vi "InstrumentSelectionByName.vi"(8 "error in (no error)":errorcluster, 9 "Verify GPIB address":bool, 11 "Instrument name IN":string) -> (0 "error out":errorcluster, 1 "Instrument name OUT":string, 2 "LCR":refnum<class "LCRControl.lvclass">, 3 "Supply":refnum<class "SupplyControl.lvclass">, 4 "Switching":refnum<class "Switching.lvclass">, 5 "Multimeter":refnum<class "MultimeterControl.lvclass">)   [LabVIEW 2018, in "InstrControl.lvclass"]
uses:
  InstrControl.lvclass
  SupplyControl/SupplyControl.lvclass
  LCRControl/LCRControl.lvclass
  MultimeterControl/MultimeterControl.lvclass
  Switching/Switching.lvclass
  ArduinoControl/ArduinoControl.lvclass
  SupplyControl/Keithley 2657/KE2657A.lvclass
  C:/Users/itk/Documents/itk-strip-sensor-qc/InstrControl/SupplyControl/SupplyControl.lvclass
  C:/Users/itk/Documents/itk-strip-sensor-qc/InstrControl/InstrControl.lvclass
  LCRControl/WK6440B/WK6440B.lvclass
  C:/Users/itk/Documents/itk-strip-sensor-qc/InstrControl/LCRControl/LCRControl.lvclass
  SupplyControl/Keithley 236 & 237/KE236.lvclass
  MultimeterControl/Keithley 2000/KE2000.lvclass
  C:/Users/itk/Documents/itk-strip-sensor-qc/InstrControl/MultimeterControl/MultimeterControl.lvclass
  Switching/Pickering/Pickering.lvclass
  C:/Users/itk/Documents/itk-strip-sensor-qc/InstrControl/Switching/Switching.lvclass
  Switching/PickeringPrague/PickeringPrague.lvclass
  InstrumentSetup.vi
  SupplyControl/Keithley 6517/KE6517.lvclass
  SupplyControl/Keithley 2410/KE2410.lvclass
  SupplyControl/Keithley 487/KE487.lvclass
  LCRControl/WK6425/WK6425.lvclass
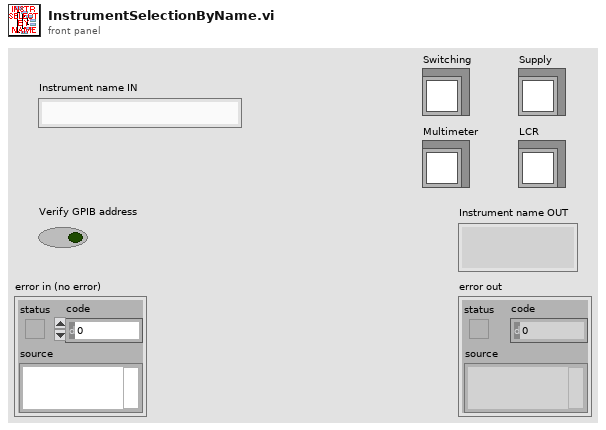
[diagram p1: front panel]
types:
  T1 = cluster{"VISA address":refnum<visa-resource-name>, "T sensor":enum16{"SHT", "DS"}, "Arduino":refnum<class "ArduinoControl.lvclass">}
  T2 = cluster{"KE 2410":cluster{"Instrument name":string, "GPIB address":string, "Instrument type":u16}, "KE 6517":cluster{"Instrument name":string, "GPIB address":string, "Instrument type":u16}, "KE 487":cluster{"Instrument name":string, "GPIB address":string, "Instrument type":u16}, "KE 487_2":cluster{"Instrument name":string, "GPIB address":string, "Instrument type":u16}, "KE 236":cluster{"Instrument name":string, "GPIB address":string, "Instrument type":u16}, "WK 6440B":cluster{"Instrument name":string, "GPIB address":string, "Instrument type":u16}, "WK 6425":cluster{"Instrument name":string, "GPIB address":string, "Instrument type":u16}, "Pickering Matrix":cluster{"Instrument name":string, "GPIB address":string, "Instrument type":u16}, "KE 2000":cluster{"Instrument name":string, "GPIB address":string, "Instrument type":u16}, "KE 2657A":cluster{"Instrument name":string, "GPIB address":string, "Instrument type":u16}, "Prague Pickering Matrix":cluster{"Instrument name":string, "GPIB address":string, "Instrument type":u16}}
  T3 = cluster{"Instrument name":string, "GPIB address":string, "Instrument type":u16}[]
  T4 = cluster{"Current Limit":sgl, "KE2410":refnum<class "KE2410.lvclass">}
  T5 = cluster{"Current Limit":u16, "KE6517":refnum<class "KE6517.lvclass">}
  T6 = cluster{"Compliance":u16, "Range:":u16, "KE487":refnum<class "KE487.lvclass">}
  T7 = cluster{"Current Limit":sgl, "Compliance":u16, "Range:":u16, "KE2657A":refnum<class "KE2657A.lvclass">}
  T8 = cluster{"current \ncompliance level":dbl, "compliance/\nmeasurement range (auto:0)":u16, "KE236":refnum<class "KE236.lvclass">}
  T9 = cluster{"RC Configuration":u16, "AC amplitude [V]":dbl, "AC frequency [Hz]":i32, "WK6440B":refnum<class "WK6440B.lvclass">}
  T10 = cluster{"RC Configuration":u16, "AC amplitude [V]":dbl, "AC frequency [Hz]":i32, "WK6425":refnum<class "WK6425.lvclass">}
  T11 = cluster{"Range":u16, "Range Value":dbl, "Function":u16, "KE2000":refnum<class "KE2000.lvclass">}
  T12 = cluster{"Matrix address":string, "Mux1 address":string, "Mux2 address":string, "Matrix used?":bool, "Pickering":refnum<class "Pickering.lvclass">, "Matrix X Channels":cluster{"Bias Supply / SMU LO":i32, "Bias Supply / SMU HI":i32, "CV Box LO":i32, "CV Box HI":i32, "CV Box LO IN":i32, "CV Box HI IN":i32, "Volt meter LO":i32, "Volt meter HI":i32, "Mux1 C1":i32, "Mux1 C2":i32, "Mux2 C1":i32, "Mux2 C2":i32}}
  T13 = cluster{"Matrix address":string, "Mux1 address":string, "Mux2 address":string, "Matrix used?":bool, "Matrix X Channels":cluster{"LCR LO":i32, "LCR HI":i32, "SMU LO":i32, "SMU HI":i32, "GND":i32}, "Matrix Y Channels":cluster{"Flying Probe":i32, "Needle":i32}, "PickeringPrague.lvclass":refnum<class "PickeringPrague.lvclass">}
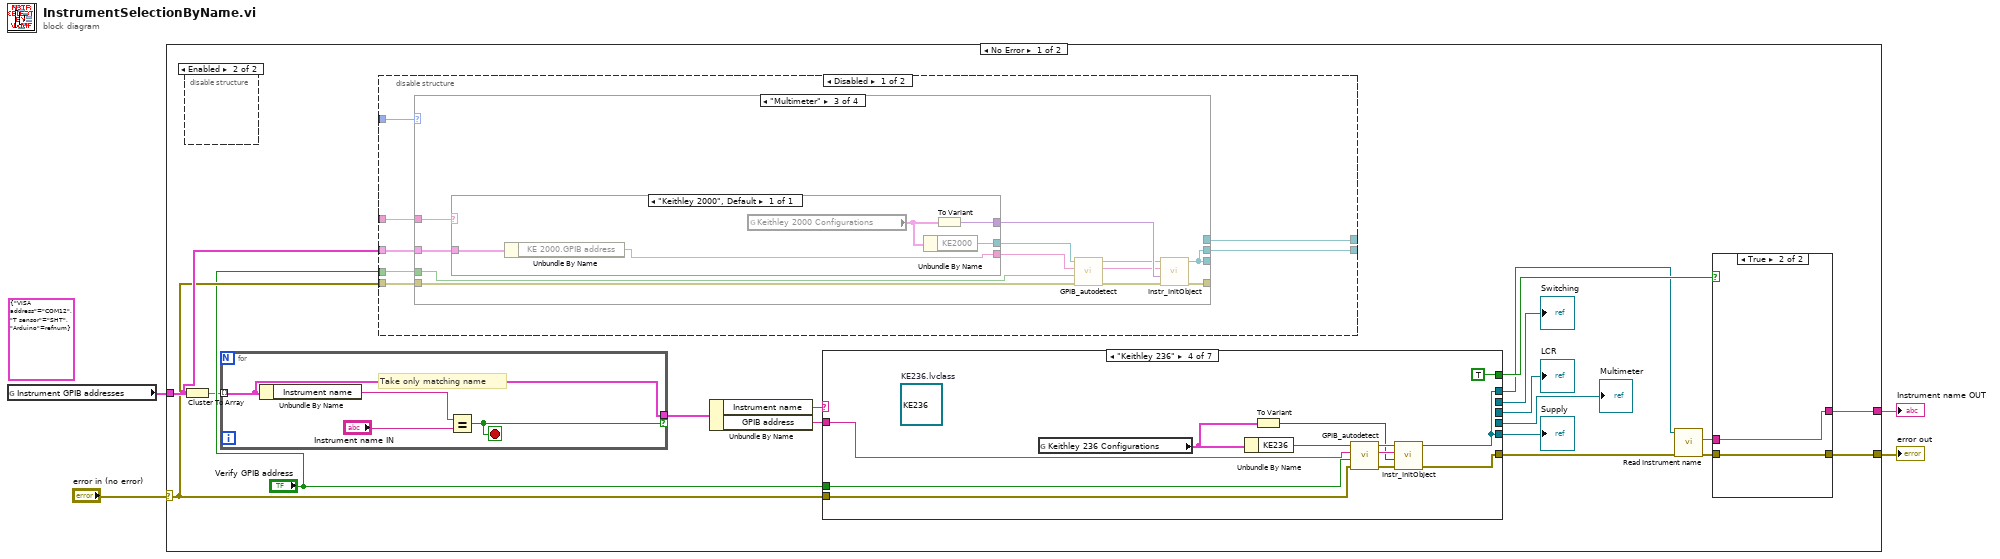
[diagram p0: block diagram]
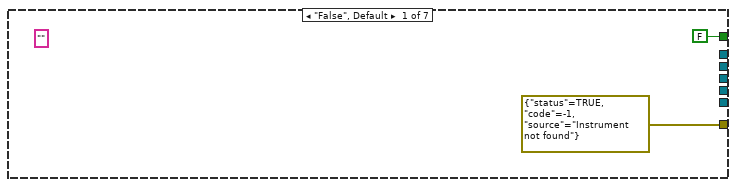
[diagram p2: hidden frame]
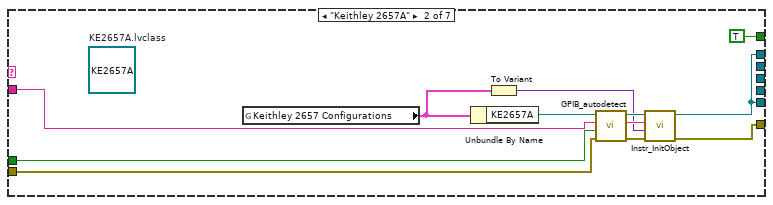
[diagram p3: hidden frame]
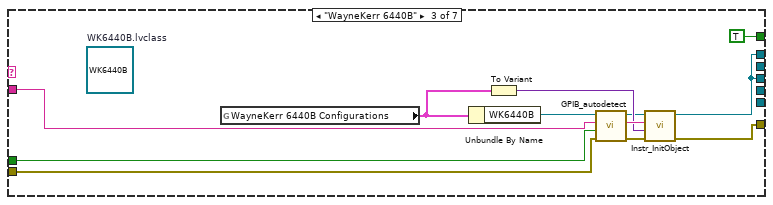
[diagram p4: hidden frame]
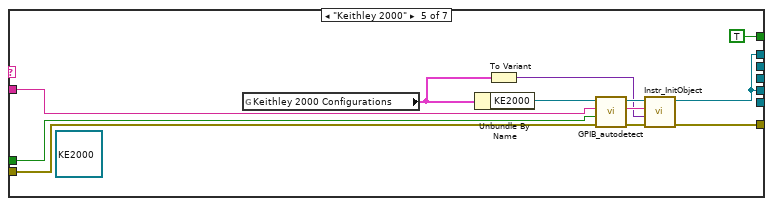
[diagram p5: hidden frame]
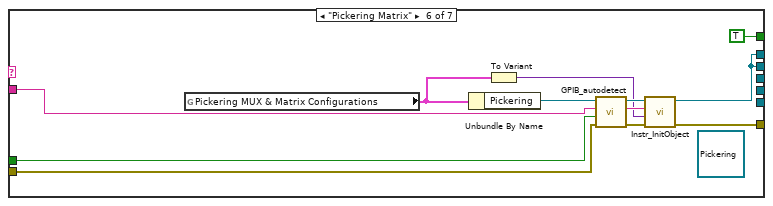
[diagram p6: hidden frame]
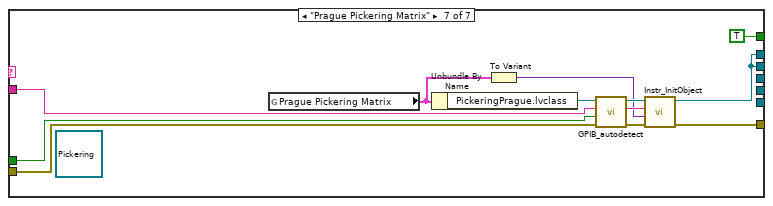
[diagram p7: hidden frame]
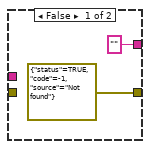
[diagram p8: hidden frame]
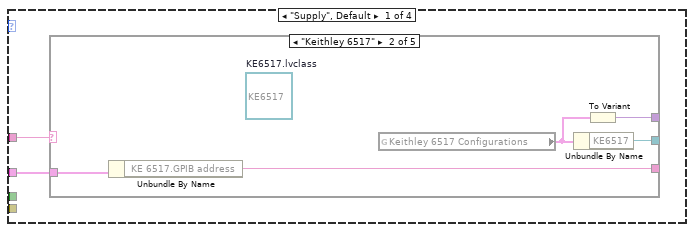
[diagram p9: hidden frame]
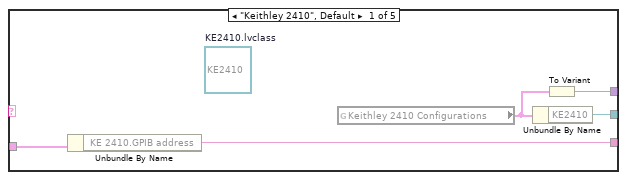
[diagram p10: hidden frame]
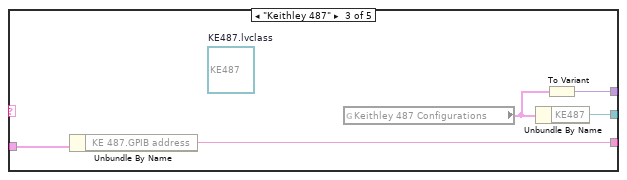
[diagram p11: hidden frame]
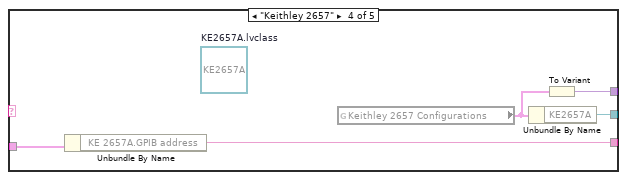
[diagram p12: hidden frame]
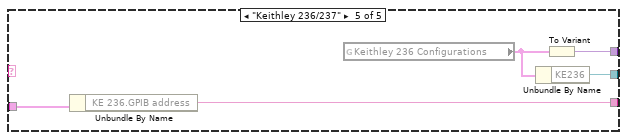
[diagram p13: hidden frame]
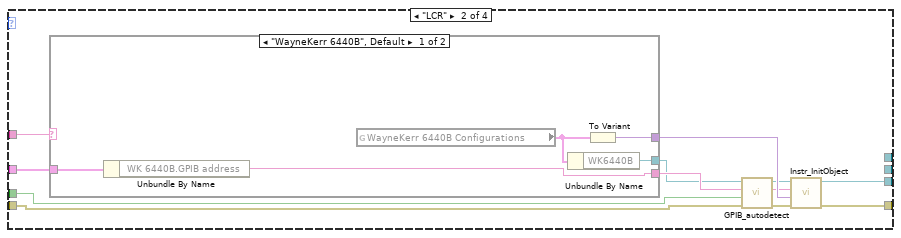
[diagram p14: hidden frame]
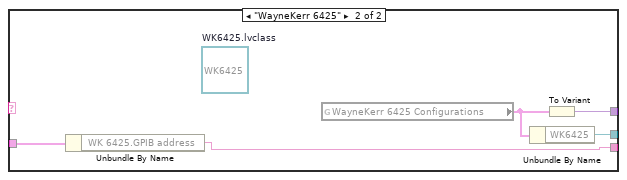
[diagram p15: hidden frame]
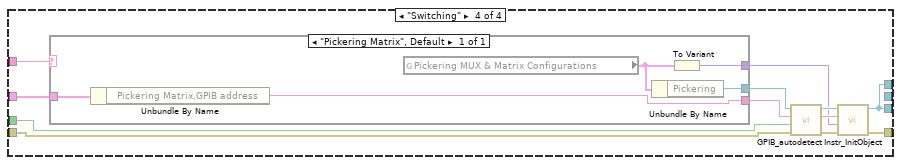
[diagram p16: hidden frame]
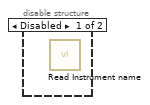
[diagram p18: hidden frame]
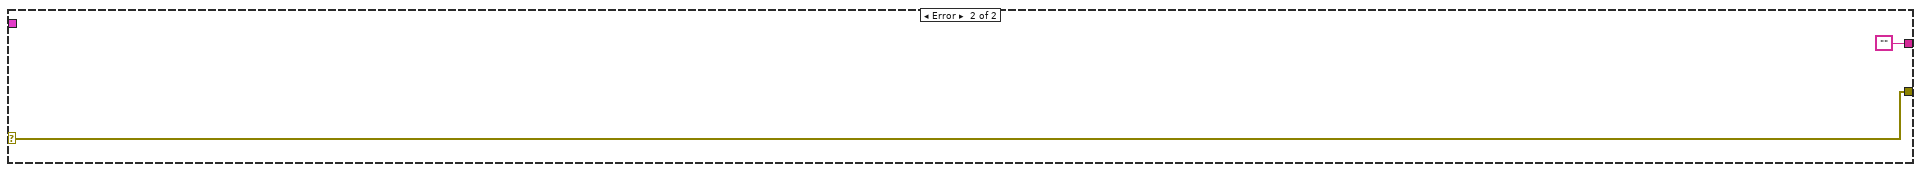
[diagram p19: hidden frame]
diagram:
  (unwired) T1 {"VISA address"="COM12", "T sensor"=enum."SHT", "Arduino"=refnum} ("Arduino Configuration")
  n1 = global read "InstrumentSetup.vi" "Instrument GPIB addresses"() -> (w2:T2)
  n2 = case shown="No Error" "error in (no error)" {
    selector: "error in (no error)" -> [w21 w196]
    tunnel: [w18 w196] -> w3
    tunnel: [w17 ""] -> w1
    tunnel: w2 -> [w22 _]
    frame No Error {
      n3 = Cluster To Array(cluster=w22) -> (array=w14:T3)
      n4 = disable-structure shown="Enabled" {
        frame Disabled {
          n5 = call-dynamic "Read Instrument name.vi"() -> ()  [unwired: 9 in, 3 out]
        }
        frame Enabled {
        }
      }
      n6 = for {
        tunnel: w14 -> [w98] mode=indexing
        tunnel: [w98] -> w13 if=w97
        stop <- w97 stop-if-true
        # "Take only matching name"
        n7 = Unbundle By Name(w98) -> ("Instrument name"=w100:string)
        n8 = Equal?(x=w100, y="Instrument name IN") -> (x = y?=w97:bool)
      }
      n9 = disable-structure shown="Disabled" {
        disable-tunnel: _ -> [w111 _]
        disable-tunnel: _ -> [w110 _]
        disable-tunnel: w22 -> [w109 _]
        disable-tunnel: w21 -> [w108 _]
        disable-tunnel: "Verify GPIB address" -> [w107 _]
        disable-tunnel: [w106 _] -> _
        disable-tunnel: [w105 _] -> _
        frame Disabled {
          n10 = case shown="\"Multimeter\"" w111 {
            tunnel: w110 -> [w113 w150 w172 w181]
            tunnel: [_ w139 w161 w178] -> _
            tunnel: w108 -> [_ w146 w163 w183]
            tunnel: [_ w149 w171 w189] -> _
            tunnel: w109 -> [w112 w148 w170 w187]
            tunnel: w107 -> [_ w140 w168 w182]
            tunnel: [_ _ _ w178] -> w106
            tunnel: [_ _ w161 _] -> w105
            frame "Supply", Default {
              n11 = case shown="\"Keithley 6517\"" w113 {
                tunnel: [w115 w119 w124 w129 w134] -> _
                tunnel: w112 -> [w118 w123 w128 w133 w138]
                tunnel: [w117 w122 w127 w132 w137] -> _
                tunnel: [w116 w121 w126 w131 w136] -> _
                frame "Keithley 2410", Default {
                  (unwired) refnum<class "KE2410.lvclass"> refnum  # KE2410.lvclass
                  n12 = Unbundle By Name(w118) -> ("KE 2410.GPIB address"=w117:string)
                  n13 = global read "InstrumentSetup.vi" "Keithley 2410 Configurations"() -> (w114:T4)
                  n14 = Unbundle By Name(w114) -> ("KE2410"=w115:refnum<class "KE2410.lvclass">)
                  n15 = To Variant(anything=w114) -> (Variant=w116:variant)
                }
                frame "Keithley 6517" {
                  (unwired) refnum<class "KE6517.lvclass"> refnum  # KE6517.lvclass
                  n16 = Unbundle By Name(w123) -> ("KE 6517.GPIB address"=w122:string)
                  n17 = global read "InstrumentSetup.vi" "Keithley 6517 Configurations"() -> (w120:T5)
                  n18 = Unbundle By Name(w120) -> ("KE6517"=w119:refnum<class "KE6517.lvclass">)
                  n19 = To Variant(anything=w120) -> (Variant=w121:variant)
                }
                frame "Keithley 487" {
                  (unwired) refnum<class "KE487.lvclass"> refnum  # KE487.lvclass
                  n20 = Unbundle By Name(w128) -> ("KE 487.GPIB address"=w127:string)
                  n21 = global read "InstrumentSetup.vi" "Keithley 487 Configurations"() -> (w125:T6)
                  n22 = Unbundle By Name(w125) -> ("KE487"=w124:refnum<class "KE487.lvclass">)
                  n23 = To Variant(anything=w125) -> (Variant=w126:variant)
                }
                frame "Keithley 2657" {
                  (unwired) refnum<class "KE2657A.lvclass"> refnum  # KE2657A.lvclass
                  n24 = Unbundle By Name(w133) -> ("KE 2657A.GPIB address"=w132:string)
                  n25 = global read "InstrumentSetup.vi" "Keithley 2657 Configurations"() -> (w130:T7)
                  n26 = Unbundle By Name(w130) -> ("KE2657A"=w129:refnum<class "KE2657A.lvclass">)
                  n27 = To Variant(anything=w130) -> (Variant=w131:variant)
                }
                frame "Keithley 236/237" {
                  n28 = Unbundle By Name(w138) -> ("KE 236.GPIB address"=w137:string)
                  n29 = global read "InstrumentSetup.vi" "Keithley 236 Configurations"() -> (w135:T8)
                  n30 = Unbundle By Name(w135) -> ("KE236"=w134:refnum<class "KE236.lvclass">)
                  n31 = To Variant(anything=w135) -> (Variant=w136:variant)
                }
              }
            }
            frame "LCR" {
              n32 = case shown="\"WayneKerr 6440B\", Default" w150 {
                tunnel: [w151 w156] -> w142
                tunnel: w148 -> [w155 w160]
                tunnel: [w154 w159] -> w144
                tunnel: [w153 w158] -> w147
                frame "WayneKerr 6440B", Default {
                  n33 = Unbundle By Name(w155) -> ("WK 6440B.GPIB address"=w154:string)
                  n34 = global read "InstrumentSetup.vi" "WayneKerr 6440B Configurations"() -> (w152:T9)
                  n35 = Unbundle By Name(w152) -> ("WK6440B"=w151:refnum<class "WK6440B.lvclass">)
                  n36 = To Variant(anything=w152) -> (Variant=w153:variant)
                }
                frame "WayneKerr 6425" {
                  (unwired) refnum<class "WK6425.lvclass"> refnum  # WK6425.lvclass
                  n37 = Unbundle By Name(w160) -> ("WK 6425.GPIB address"=w159:string)
                  n38 = global read "InstrumentSetup.vi" "WayneKerr 6425 Configurations"() -> (w157:T10)
                  n39 = Unbundle By Name(w157) -> ("WK6425"=w156:refnum<class "WK6425.lvclass">)
                  n40 = To Variant(anything=w157) -> (Variant=w158:variant)
                }
              }
              n41 = call-dynamic "GPIB_autodetect.vi"("error in (no error)"=w146, "Verify GPIB address"=w140, "Instrument GPIB address in"=w144, "InstrControl in"=w142) -> ("error out"=w145:errorcluster, "Instrument GPIB address"=w143:string, "InstrControl out"=w141:refnum<class "LCRControl.lvclass">)  [unwired: 5 in]
              n42 = call-dynamic "Instr_InitObject.vi"("error in (no error)"=w145, "Instrument Configuration"=w147, "GPIB Address"=w143, "LCRControl in"=w141) -> ("error out"=w149:errorcluster, "LCRControl out"=w139:refnum<class "LCRControl.lvclass">)  [unwired: 6 in]
            }
            frame "Multimeter" {
              n43 = case shown="\"Keithley 2000\", Default" w172 {
                tunnel: [w173] -> w164
                tunnel: w170 -> [w177]
                tunnel: [w176] -> w167
                tunnel: [w175] -> w169
                frame "Keithley 2000", Default {
                  n44 = Unbundle By Name(w177) -> ("KE 2000.GPIB address"=w176:string)
                  n45 = global read "InstrumentSetup.vi" "Keithley 2000 Configurations"() -> (w174:T11)
                  n46 = Unbundle By Name(w174) -> ("KE2000"=w173:refnum<class "KE2000.lvclass">)
                  n47 = To Variant(anything=w174) -> (Variant=w175:variant)
                }
              }
              n48 = call-dynamic "GPIB_autodetect.vi"("error in (no error)"=w163, "Verify GPIB address"=w168, "Instrument GPIB address in"=w167, "InstrControl in"=w164) -> ("error out"=w162:errorcluster, "Instrument GPIB address"=w166:string, "InstrControl out"=w165:refnum<class "KE2000.lvclass">)  [unwired: 5 in]
              n49 = call-dynamic "Instr_InitObject.vi"("error in (no error)"=w162, "Instrument Configuration"=w169, "GPIB Address"=w166, "KE2000 in"=w165) -> ("error out"=w171:errorcluster, "KE2000 out"=w161:refnum<class "KE2000.lvclass">)  [unwired: 6 in]
            }
            frame "Switching" {
              n50 = case shown="\"Pickering Matrix\", Default" w181 {
                tunnel: w187 -> [w194]
                tunnel: [w193] -> w186
                tunnel: [w191] -> w180
                tunnel: [w190] -> w179
                frame "Pickering Matrix", Default {
                  n51 = Unbundle By Name(w194) -> ("Pickering Matrix.GPIB address"=w193:string)
                  n52 = global read "InstrumentSetup.vi" "Pickering MUX & Matrix Configurations"() -> (w192:T12)
                  n53 = Unbundle By Name(w192) -> ("Pickering"=w190:refnum<class "Pickering.lvclass">)
                  n54 = To Variant(anything=w192) -> (Variant=w191:variant)
                }
              }
              n55 = call-dynamic "GPIB_autodetect.vi"("error in (no error)"=w183, "Verify GPIB address"=w182, "Instrument GPIB address in"=w186, "InstrControl in"=w179) -> ("error out"=w185:errorcluster, "Instrument GPIB address"=w184:string, "InstrControl out"=w188:refnum<class "Pickering.lvclass">)  [unwired: 5 in]
              n56 = call-dynamic "Instr_InitObject.vi"("error in (no error)"=w185, "Instrument Configuration"=w180, "GPIB Address"=w184, "Pickering in"=w188) -> ("error out"=w189:errorcluster, "Pickering out"=w178:refnum<class "Pickering.lvclass">)  [unwired: 6 in]
            }
          }
        }
        frame Enabled {
        }
      }
      n57 = Unbundle By Name(w13) -> ("Instrument name"=w12:string, "GPIB address"=w11:string)
      n58 = case shown="\"Keithley 236\"" w12 {
        tunnel: w11 -> [_ w29 w45 w53 w65 w77 w89]
        tunnel: w21 -> [_ w32 w47 w56 w68 w80 w92]
        tunnel: "Verify GPIB address" -> [_ w31 w46 w55 w67 w79 w91]
        tunnel: [_ w26 _ w50 _ _ _] -> w8
        tunnel: [FALSE TRUE TRUE TRUE TRUE TRUE TRUE] -> w19
        tunnel: [_ _ _ _ _ w73 w85] -> w9
        tunnel: [_ _ w38 _ _ _ _] -> w10
        tunnel: [_ w26 w38 w50 w61 w73 w85] -> w6
        tunnel: [errorcluster {"status"=TRUE, "code"=-1, "source"="Instrument not found"} ("error out") w25 w37 w49 w62 w74 w86] -> w7
        tunnel: [_ _ _ _ w61 _ _] -> w5
        frame "False", Default {
          (unwired) "" ("Instrument name")
        }
        frame "Keithley 2657A" {
          (unwired) refnum<class "KE2657A.lvclass"> refnum  # KE2657A.lvclass
          n59 = global read "InstrumentSetup.vi" "Keithley 2657 Configurations"() -> (w36:T7)
          n60 = Unbundle By Name(w36) -> ("KE2657A"=w30:refnum<class "KE2657A.lvclass">)
          n61 = To Variant(anything=w36) -> (Variant=w28:variant)
          n62 = call-dynamic "GPIB_autodetect.vi"("error in (no error)"=w32, "Verify GPIB address"=w31, "Instrument GPIB address in"=w29, "InstrControl in"=w30) -> ("error out"=w35:errorcluster, "Instrument GPIB address"=w33:string, "InstrControl out"=w34:refnum<class "KE2657A.lvclass">)  [unwired: 5 in]
          n63 = call-dynamic "Instr_InitObject.vi"("error in (no error)"=w35, "Instrument Configuration"=w28, "GPIB address"=w33, "KE2657A in"=w34) -> ("error out"=w25:errorcluster, "KE2657A out"=w26:refnum<class "KE2657A.lvclass">)  [unwired: 6 in]
        }
        frame "WayneKerr 6440B" {
          (unwired) refnum<class "WK6440B.lvclass"> refnum  # WK6440B.lvclass
          n64 = global read "InstrumentSetup.vi" "WayneKerr 6440B Configurations"() -> (w48:T9)
          n65 = Unbundle By Name(w48) -> ("WK6440B"=w43:refnum<class "WK6440B.lvclass">)
          n66 = To Variant(anything=w48) -> (Variant=w41:variant)
          n67 = call-dynamic "GPIB_autodetect.vi"("error in (no error)"=w47, "Verify GPIB address"=w46, "Instrument GPIB address in"=w45, "InstrControl in"=w43) -> ("error out"=w40:errorcluster, "Instrument GPIB address"=w42:string, "InstrControl out"=w39:refnum<class "WK6440B.lvclass">)  [unwired: 5 in]
          n68 = call-dynamic "Instr_InitObject.vi"("error in (no error)"=w40, "Instrument Configuration"=w41, "GPIB Address"=w42, "WK6440B in"=w39) -> ("error out"=w37:errorcluster, "WK6440B out"=w38:refnum<class "WK6440B.lvclass">)  [unwired: 6 in]
        }
        frame "Keithley 236" {
          (unwired) refnum<class "KE236.lvclass"> refnum  # KE236.lvclass
          n69 = global read "InstrumentSetup.vi" "Keithley 236 Configurations"() -> (w60:T8)
          n70 = Unbundle By Name(w60) -> ("KE236"=w54:refnum<class "KE236.lvclass">)
          n71 = To Variant(anything=w60) -> (Variant=w52:variant)
          n72 = call-dynamic "GPIB_autodetect.vi"("error in (no error)"=w56, "Verify GPIB address"=w55, "Instrument GPIB address in"=w53, "KE236 in"=w54) -> ("error out"=w59:errorcluster, "Instrument GPIB address"=w57:string, "KE236 out"=w58:refnum<class "KE236.lvclass">)  [unwired: 5 in]
          n73 = call-dynamic "Instr_InitObject.vi"("error in (no error)"=w59, "Instrument Configuration"=w52, "GPIB address"=w57, "KE236 in"=w58) -> ("error out"=w49:errorcluster, "KE236 out"=w50:refnum<class "KE236.lvclass">)  [unwired: 6 in]
        }
        frame "Keithley 2000" {
          (unwired) refnum<class "KE2000.lvclass"> refnum ("KE2000.lvclass")
          n74 = global read "InstrumentSetup.vi" "Keithley 2000 Configurations"() -> (w72:T11)
          n75 = Unbundle By Name(w72) -> ("KE2000"=w66:refnum<class "KE2000.lvclass">)
          n76 = To Variant(anything=w72) -> (Variant=w64:variant)
          n77 = call-dynamic "GPIB_autodetect.vi"("error in (no error)"=w68, "Verify GPIB address"=w67, "Instrument GPIB address in"=w65, "InstrControl in"=w66) -> ("error out"=w71:errorcluster, "Instrument GPIB address"=w69:string, "InstrControl out"=w70:refnum<class "KE2000.lvclass">)  [unwired: 5 in]
          n78 = call-dynamic "Instr_InitObject.vi"("error in (no error)"=w71, "Instrument Configuration"=w64, "GPIB Address"=w69, "KE2000 in"=w70) -> ("error out"=w62:errorcluster, "KE2000 out"=w61:refnum<class "KE2000.lvclass">)  [unwired: 6 in]
        }
        frame "Pickering Matrix" {
          (unwired) refnum<class "Pickering.lvclass"> refnum ("Pickering")
          n79 = global read "InstrumentSetup.vi" "Pickering MUX & Matrix Configurations"() -> (w84:T12)
          n80 = Unbundle By Name(w84) -> ("Pickering"=w78:refnum<class "Pickering.lvclass">)
          n81 = To Variant(anything=w84) -> (Variant=w76:variant)
          n82 = call-dynamic "GPIB_autodetect.vi"("error in (no error)"=w80, "Verify GPIB address"=w79, "Instrument GPIB address in"=w77, "InstrControl in"=w78) -> ("error out"=w83:errorcluster, "Instrument GPIB address"=w81:string, "InstrControl out"=w82:refnum<class "Pickering.lvclass">)  [unwired: 5 in]
          n83 = call-dynamic "Instr_InitObject.vi"("error in (no error)"=w83, "Instrument Configuration"=w76, "GPIB Address"=w81, "Pickering in"=w82) -> ("error out"=w74:errorcluster, "Pickering out"=w73:refnum<class "Pickering.lvclass">)  [unwired: 6 in]
        }
        frame "Prague Pickering Matrix" {
          (unwired) refnum<class "Pickering.lvclass"> refnum ("Pickering")
          n84 = global read "InstrumentSetup.vi" "Prague Pickering Matrix"() -> (w96:T13)
          n85 = Unbundle By Name(w96) -> ("PickeringPrague.lvclass"=w90:refnum<class "PickeringPrague.lvclass">)
          n86 = To Variant(anything=w96) -> (Variant=w88:variant)
          n87 = call-dynamic "GPIB_autodetect.vi"("error in (no error)"=w92, "Verify GPIB address"=w91, "Instrument GPIB address in"=w89, "InstrControl in"=w90) -> ("error out"=w95:errorcluster, "Instrument GPIB address"=w93:string, "InstrControl out"=w94:refnum<class "PickeringPrague.lvclass">)  [unwired: 5 in]
          n88 = call-dynamic "Instr_InitObject.vi"("error in (no error)"=w95, "Instrument Configuration"=w88, "GPIB Address"=w93, "Pickering in"=w94) -> ("error out"=w86:errorcluster, "Pickering out"=w85:refnum<class "PickeringPrague.lvclass">)  [unwired: 6 in]
        }
      }
      "Supply" <- w8
      "LCR" <- w10
      "Switching" <- w9
      "Multimeter" <- w5
      n89 = call-dynamic "Read Instrument name.vi"("error in (no error)"=w7, "InstControl in"=w6) -> ("error out"=w15:errorcluster, "Instrument name"=w16:string)  [unwired: 7 in, 1 out]
      n90 = case shown="True" w19 {
        tunnel: [errorcluster {"status"=TRUE, "code"=-1, "source"="Not found"} ("error IO") w103] -> w18
        tunnel: ["" ("Instrument name") w104] -> w17
        tunnel: w16 -> [_ w104]
        tunnel: w15 -> [_ w103]
        frame False {
        }
        frame True {
        }
      }
    }
    frame Error {
    }
  }
  "error out" <- w3
  "Instrument name OUT" <- w1
